vi "Enum to Num.vi"(1 "Command":T1(ring)) -> (0 "Std Command":i32=6)   [LabVIEW 2015]
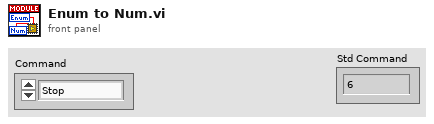
[diagram p1: front panel]
types:
  T1 = enum16{"Stop", "LED", "Front", "Back", "Left", "Right"}
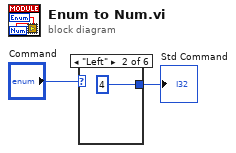
[diagram p0: block diagram]
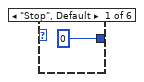
[diagram p2: hidden frame]
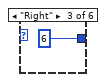
[diagram p3: hidden frame]
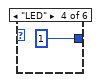
[diagram p4: hidden frame]
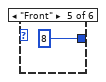
[diagram p5: hidden frame]
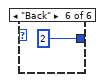
[diagram p6: hidden frame]
diagram:
  n1 = case shown="\"Left\"" "Command" {
    tunnel: [0 4 6 1 8 2] -> w1
    frame "Stop", Default {
    }
    frame "Left" {
    }
    frame "Right" {
    }
    frame "LED" {
    }
    frame "Front" {
    }
    frame "Back" {
    }
  }
  "Std Command" <- w1
